vi "Resampling example.vi"() -> ()   [LabVIEW 2018]
uses:
  <vilib>/measure/maresamp.llb/Resample Waveform (single shot).vi
  <vilib>/measure/NI_MABase.lvlib
  <vilib>/measure/NI_MAPro.lvlib
panel:
  out "Number of samples":dbl format="%#_13g"
  out "Sampling Freq":dbl format="%#_13g"
  out "Resampling Frequency":dbl format="%#_13g"
  in  "amplitude":dbl=1.0 format="%0.2p"
  in  "frequency":dbl=10.0 format="%0.2p"
  out "Original":waveform(dbl)(graph)
  out "Resample":waveform(dbl)(graph)
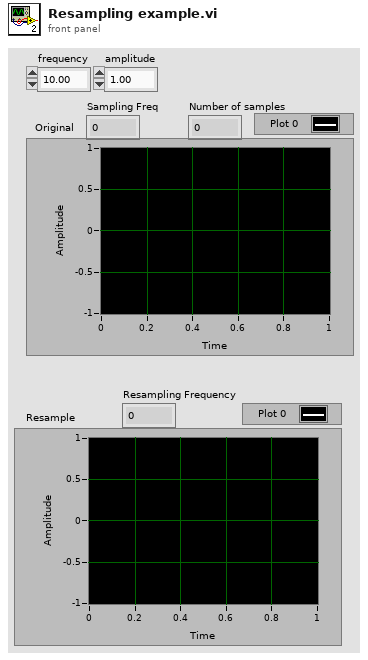
[diagram p1: front panel]
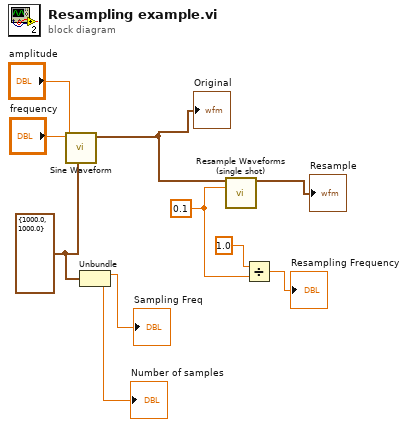
[diagram p0: block diagram]
diagram:
  w3 = cluster{"Fs":dbl, "#s":dbl} {"Fs"=1000.0, "#s"=1000.0} ("sampling info")
  w4 = 0.1 ("dt")
  n1 = call <vilib>:"Sine Waveform.vi"("sampling info"=w3, "amplitude"="amplitude", "frequency"="frequency") -> ("signal out"=w8:waveform(dbl))  [unwired: 7 in, 1 out]
  "Original" <- w8
  n2 = Unbundle(w3) -> ("Fs"=→"Sampling Freq":dbl, "#s"=→"Number of samples":dbl)
  n3 = call-poly <vilib>:"Resample Waveforms (single shot).vi"("waveform in"=w8, "dt"=w4) -> ("resampled waveform out"=→"Resample":waveform(dbl))  [unwired: 10 in, 3 out]
  n4 = Divide(x=1.0, y=w4) -> (x/y=→"Resampling Frequency":dbl)
